vi "pumpSwitch.vi"(8 "error in (no error)":errorcluster, 10 "Sensors":refnum<class "Sensor.lvclass">[](array[class]), 11 "Pump in":refnum<class "Pump.lvclass">) -> (0 "error out":errorcluster, 3 "Pump out":refnum<class "Pump.lvclass">)   [LabVIEW 2020, in "Pump.lvclass"]
uses:
  Pump.lvclass
  Sensor Class/Sensor.lvclass
  Pump.lvclass/Pump.ctl
  Sensor Class/Sensor.lvclass/Sensor.ctl
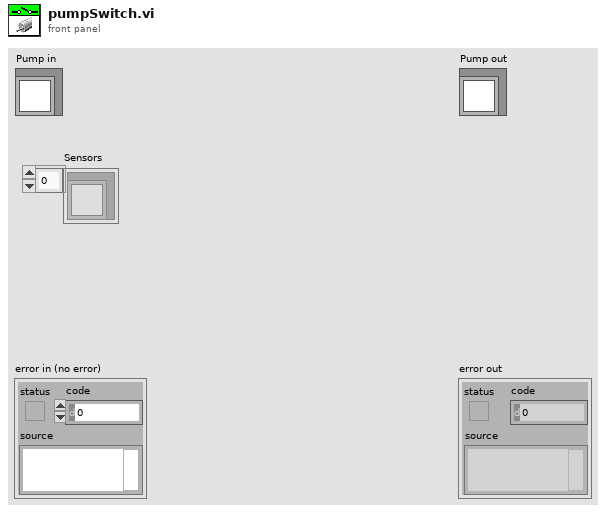
[diagram p1: front panel]
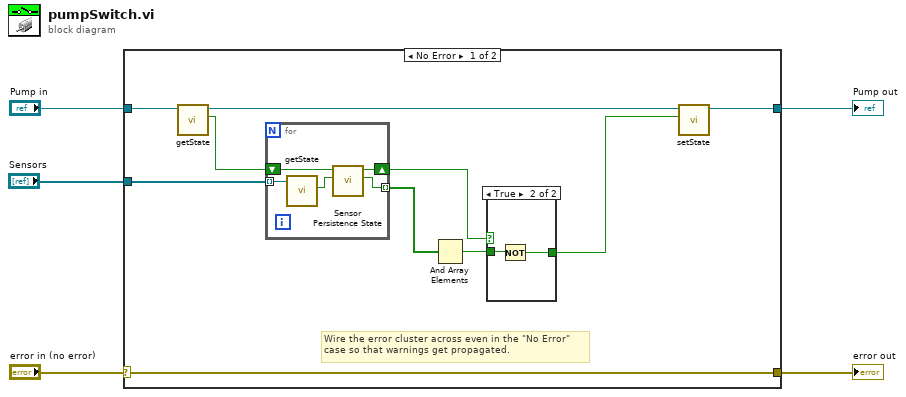
[diagram p0: block diagram]
diagram:
  n1 = case shown="No Error" "error in (no error)" {
    selector: "error in (no error)" -> [w15 w25]
    tunnel: [w15 w25] -> w4
    tunnel: [w11 w24] -> w2
    tunnel: "Pump in" -> [w13 w24]
    tunnel: "Sensors" -> [w14 _]
    frame No Error {
      # "Wire the error cluster across even in the \"No Error\"\ncase so that warnings get propagated."
      n2 = call "getState.vi"("Pump in"=w13) -> ("state"=w10:bool, "Pump out"=w12:refnum<class "Pump.lvclass">)  [unwired: 8 in, 1 out]
      n3 = for {
        tunnel: w14 -> [w23] mode=indexing
        tunnel: [w21] -> w9 mode=indexing
        shift-right: [w19] -> w6
        shift-left: w10 -> [w20]
        n4 = call "getState.vi"("Sensor in"=w23) -> ("State"=w22:bool)  [unwired: 8 in, 2 out]
        n5 = call "Sensor Persistence State.vi"("Sensor"=w22, "Pump State in"=w20) -> ("Persistent State"=w21:bool, "Pump State out"=w19:bool)  [unwired: 8 in]
      }
      n6 = And Array Elements(Boolean array=w9) -> (logical AND=w8:bool)
      n7 = case shown="True" w6 {
        tunnel: w8 -> [w16 w18]
        tunnel: [w16 w17] -> w7
        frame False {
        }
        frame True {
          n8 = Not(x=w18) -> (.not. x?=w17:bool)
        }
      }
      n9 = call "setState.vi"("state"=w7, "Pump in"=w12) -> ("Pump out"=w11:refnum<class "Pump.lvclass">)  [unwired: 8 in, 1 out]
    }
    frame Error {
    }
  }
  "error out" <- w4
  "Pump out" <- w2
